vi "Stop Core.vi"(10 "final error code":i32, 11 "Logger in":refnum<class "Logger.lvclass">) -> (3 "Logger out":refnum<class "Logger.lvclass">)   [LabVIEW 2017, in "Logger.lvlib" / "Logger.lvclass"]
doc: "(<B>Filename</B>: Actor Framework.lvlib:Actor.lvclass:Stop Core.vi)\n\nDefines what the actor does before it stops. Use the <B>final error code</B> input to determine whether the actor shut down in response to an error.\n\nBy default, this method does nothing. A descendant class may override it to define behavior, such as shutting down any processes the actor initiated in its override of the Actor Core method."
uses:
  Logger.lvclass
  Logger.lvclass/Logger.ctl
  <vilib>/ActorFramework/Actor/Actor.lvclass
  <vilib>/Skyline/Configuration/Configuration AMQP_class/NI Skyline Configuration AMQP.lvclass
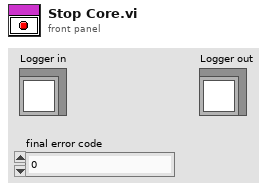
[diagram p1: front panel]
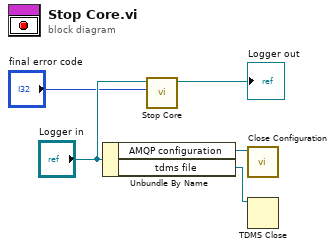
[diagram p0: block diagram]
diagram:
  n1 = Unbundle By Name("Logger in") -> ("AMQP configuration"=w3:refnum<class "NI Skyline Configuration AMQP.lvclass">, "tdms file"=w1:refnum<k34>)
  n2 = call-parent "Stop Core.vi"("final error code"="final error code", "Actor in"="Logger in") -> ("Actor out"=→"Logger out":refnum<class "Logger.lvclass">)  [unwired: 9 in]
  n3 = call-dynamic "Close Configuration.vi"("AMQP configuration in"=w3) -> ()  [unwired: 10 in, 1 out]
  n4 = TDMS Close(11:w1) -> ()  [unwired: 1 in, 2 out]
